vi "Set Pin Map ID.vi"(8 "error in":errorcluster, 10 "pin_map_id":string, 11 "Sequence Context":refnum<k7>) -> (0 "error out":errorcluster)   [LabVIEW 2020, in "NIFgenStandardFunction.lvlib"]
uses:
  NIFgenStandardFunction.lvlib
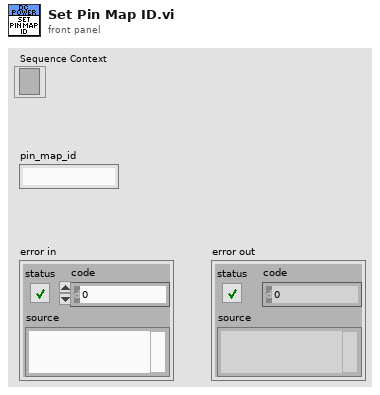
[diagram p1: front panel]
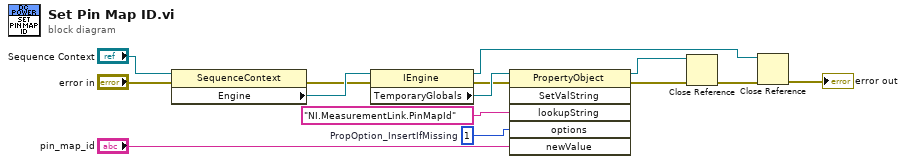
[diagram p0: block diagram]
diagram:
  w1 = 1  # PropOption_InsertIfMissing
  n1 = property class="SequenceContext"(reference="Sequence Context", error in="error in") -> (error out=w5:errorcluster, "Engine"=w7:refnum<k7>)  [unwired: 1 out]
  n2 = property class="IEngine"(reference=w7, error in=w5) -> (reference out=w12:refnum<k7>, error out=w3:errorcluster, "TemporaryGlobals"=w8:refnum<k7>)
  n3 = invoke class="PropertyObject" method="SetValString"(reference=w8, error in=w3, "lookupString"="NI.MeasurementLink.PinMapId", "options"=w1, "newValue"="pin_map_id") -> (reference out=w10:refnum<k7>, error out=w11:errorcluster)  [unwired: 1 in, 4 out]
  n4 = Close Reference(reference=w10, error in (no error)=w11) -> (error out=w13:errorcluster)
  n5 = Close Reference(reference=w12, error in (no error)=w13) -> (error out=→"error out":errorcluster)
